vi "compute_zernike_coeffs_starter.vi"() -> ()   [LabVIEW 2020]
uses:
  HasoSlopes.lvclass
  Pupil.lvclass
  ModalCoef.lvclass
panel:
  out "Zernike pupil":i32[][](graph)
  out "Measured pupil":i32[][](graph)
  out "Zernike Coefficients":sgl[](graph)
  in  "Haso slopes file name":string="Data\\data_phase_computation.has"
  out "error out":errorcluster
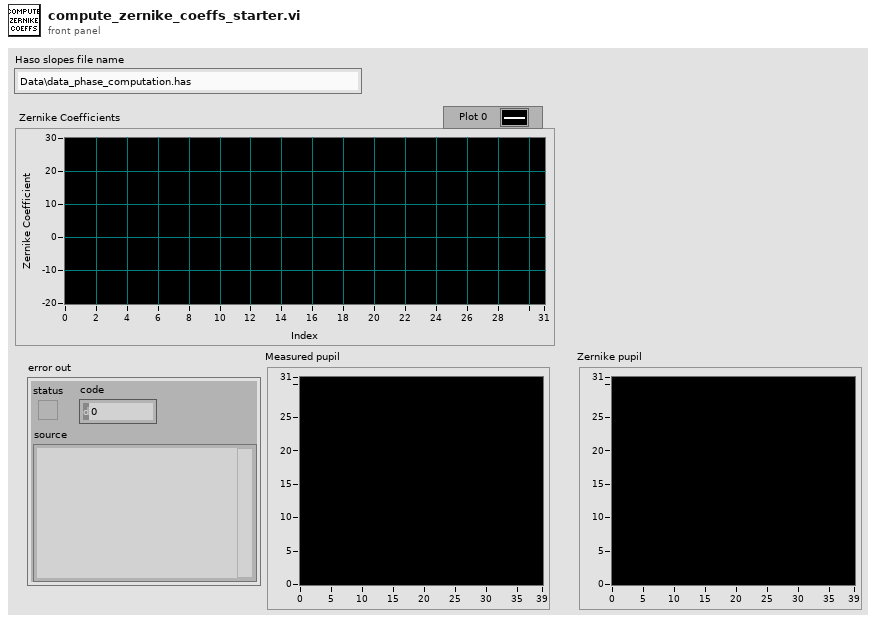
[diagram p1: front panel]
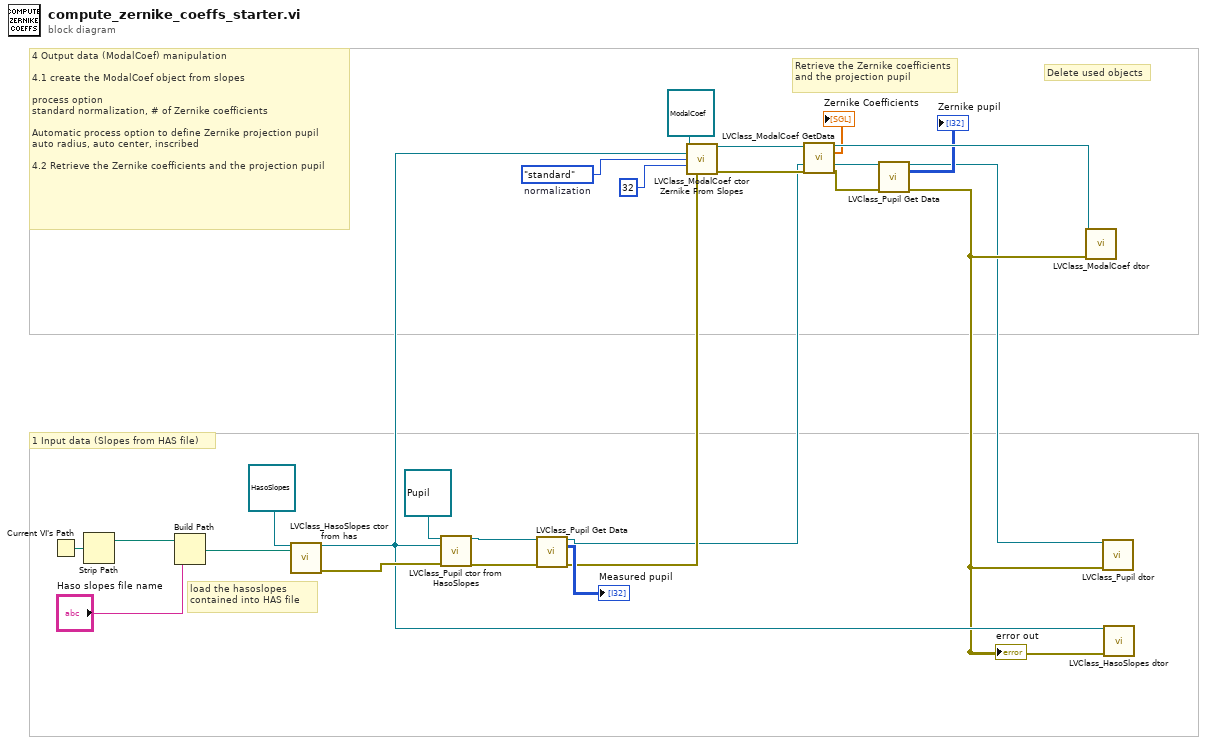
[diagram p0: block diagram]
diagram:
  w7 = enum16{"standard", "rms"}."standard"  # normalization
  # "4 Output data (ModalCoef) manipulation\n\n4.1 create the ModalCoef object from slopes\n\nprocess option\nstandard normalization, # of Zernike coefficients\n\nAutomatic process option to define Zernike projection pupil\nauto radius, auto center, inscribed\n\n4.2 Retrieve the Zernike coefficients and the projection pupil"
  # "Retrieve the Zernike coefficients and the projection pupil"
  # "1 Input data (Slopes from HAS file)"
  # "Delete used objects"
  # "load the hasoslopes\ncontained into HAS file"
  n1 = Current VI's Path() -> (path=w22:path)
  n2 = Strip Path(path=w22) -> (stripped path=w19:path)  [unwired: 1 out]
  n3 = Build Path(base path=w19, name or relative path="Haso slopes file name") -> (appended path=w20:path)
  n4 = call "LVClass_HasoSlopes ctor from has.vi"("HasoSlopes in"=refnum<class "HasoSlopes.lvclass"> refnum, ".has path"=w20) -> ("HasoSlopes out"=w9:refnum<class "HasoSlopes.lvclass">, "error out"=w18:errorcluster)  [unwired: 12 in]
  n5 = call "LVClass_Pupil ctor from HasoSlopes.vi"("Pupil in"=refnum<class "Pupil.lvclass"> refnum, "HasoSlopes.lvclass"=w9, "error in (no error)"=w18) -> ("Pupil out"=w14:refnum<class "Pupil.lvclass">, "error out"=w13:errorcluster)  [unwired: 11 in]
  n6 = call "LVClass_Pupil Get Data.vi"("Pupil in"=w14, "error in (no error)"=w13) -> ("Pupil out"=w2:refnum<class "Pupil.lvclass">, "Data"=→"Measured pupil":i32[][], "error out"=w12:errorcluster)  [unwired: 11 in]
  n7 = call "LVClass_ModalCoef ctor Zernike From Slopes.vi"("ModalCoef in"=refnum<class "ModalCoef.lvclass"> refnum, "HasoSlopes"=w9, "normalization"=w7, "nb_coefs"=u32 32, "error in (no error)"=w12) -> ("ModalCoef out"=w11:refnum<class "ModalCoef.lvclass">, "error out"=w10:errorcluster)  [unwired: 9 in]
  n8 = call "LVClass_ModalCoef GetData.vi"("ModalCoef in"=w11, "Pupil.lvclass"=w2, "error in (no error)"=w10) -> ("ModalCoef out"=w23:refnum<class "ModalCoef.lvclass">, "coef"=→"Zernike Coefficients":sgl[], "Pupil.lvclass (dup)"=w6:refnum<class "Pupil.lvclass">, "error out"=w5:errorcluster)  [unwired: 8 in, 1 out]
  n9 = call "LVClass_Pupil Get Data.vi"("Pupil in"=w6, "error in (no error)"=w5) -> ("Pupil out"=w1:refnum<class "Pupil.lvclass">, "Data"=→"Zernike pupil":i32[][], "error out"=w4:errorcluster)  [unwired: 11 in]
  "error out" <- w4
  n10 = call "LVClass_ModalCoef dtor.vi"("ModalCoef in"=w23, "error in (no error)"=w4) -> ()  [unwired: 12 in, 2 out]
  n11 = call "LVClass_Pupil dtor.vi"("Pupil in"=w1, "error in (no error)"=w4) -> ()  [unwired: 12 in, 2 out]
  n12 = call "LVClass_HasoSlopes dtor.vi"("HasoSlopes in"=w9, "error in (no error)"=w4) -> ()  [unwired: 12 in, 2 out]
